vi "get shm direction from lines.vi"(8 "error in":errorcluster, 11 "Lines in":T1[](array[typedef])) -> (0 "error out":errorcluster, 1 "all same direction?":bool, 2 "direction string":string, 3 "Lines out":T1[](array[typedef]))   [LabVIEW 2014, in "Shared Memory configuration.lvclass"]
uses:
  Shared Memory configuration.lvclass
  Line.ctl
  <vilib>/NI/Tag Bus Module Framework/channel/TBM channel.lvclass
  <vilib>/NI/Tag Bus Module Framework/channel/TBM channel.lvclass/TBM channel.ctl
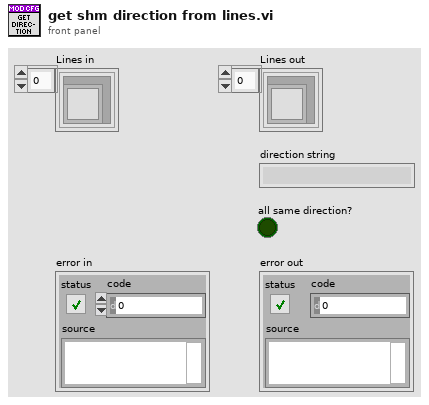
[diagram p1: front panel]
types:
  T1 = typedef "Shared Memory configuration.lvclass/Line.ctl" = cluster{"channel":refnum<class "TBM channel.lvclass">}
  T2 = typedef "TBM channel.lvclass/channel classification.ctl" = enum16{"input data", "output data", "processing parameter", "processing result"}
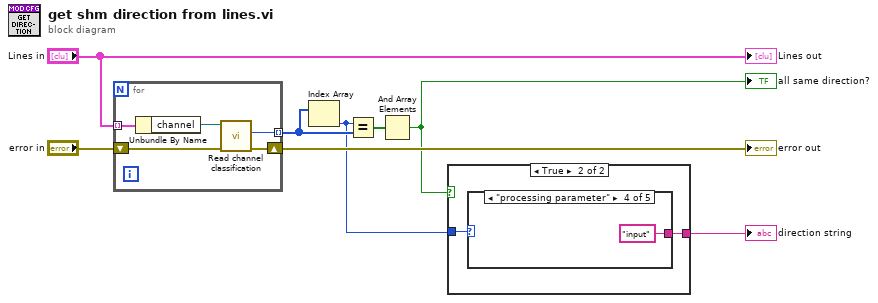
[diagram p0: block diagram]
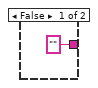
[diagram p2: hidden frame]
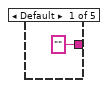
[diagram p3: hidden frame]
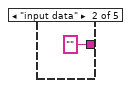
[diagram p4: hidden frame]
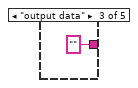
[diagram p5: hidden frame]
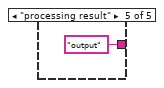
[diagram p6: hidden frame]
diagram:
  n1 = for {
    tunnel: "Lines in" -> [w13] mode=indexing
    tunnel: [w11] -> w6 mode=indexing
    shift-right: [w10] -> w4
    shift-left: "error in" -> [w9]
    n2 = Unbundle By Name(w13) -> ("channel"=w12:refnum<class "TBM channel.lvclass">)
    n3 = call <vilib>:"Read channel classification.vi"("error in"=w9, "channel in"=w12) -> ("error out"=w10:errorcluster, "channel classification"=w11:T2)  [unwired: 7 in, 1 out]
  }
  "error out" <- w4
  n4 = Index Array(array=w6) -> (element=w2:T2)  [unwired: 1 in]
  n5 = Equal?(x=w2, y=w6) -> (x = y?=w5:bool[])
  n6 = And Array Elements(Boolean array=w5) -> (logical AND=w3:bool)
  "all same direction?" <- w3
  n7 = case shown="True" w3 {
    tunnel: w2 -> [_ w16]
    tunnel: ["" w15] -> w1
    frame False {
    }
    frame True {
      n8 = case shown="\"processing parameter\"" w16 {
        tunnel: ["" "" "" "input" "output"] -> w15
        frame Default {
        }
        frame "input data" {
        }
        frame "output data" {
        }
        frame "processing parameter" {
        }
        frame "processing result" {
        }
      }
    }
  }
  "direction string" <- w1
  "Lines out" <- "Lines in"
